vi "Teleop.vi"(10 "Match Info":T1={"Autonomous Elapsed Seconds"=0.0, "TeleOp Elapsed Seconds"=0.0, "Disabled Elapsed Seconds"=0.0, "Visited Autonomous"=FALSE, "Visited TeleOp"=FALSE, "Visited Disabled"=FALSE, "Autonomous Settings"={"Autonomous Style"=enum."Independent", "VI Refnum"=refnum}}, 11 "Call Context":T2) -> ()   [LabVIEW 2016]
doc: "This VI is called for each TeleOp packet received from the DS where the robot is not disabled. It is often used to read from the joysticks and update I/O or to update setpoints for timed control loops. It should complete and return within 20 milliseconds or it may miss DS packets."
uses:
  <vilib>/Rock Robotics/WPI/DriverStation/WPI_DriverStationDerivedRobotMode.ctl
  <vilib>/Rock Robotics/WPI/DriverStation/WPI_DriverStationMatch Info.ctl
  Refname/Controllers.ctl
  Refname/Motors.ctl
  Refname/Refname to String (Controllers).vi
  <vilib>/Rock Robotics/WPI/Utilities/WPI_GetSetVariantRefNum.vi
  Robot Global Data.vi
panel:
  out "Final Offsets":dbl[](array[numeric])
  out "error constant":errorcluster
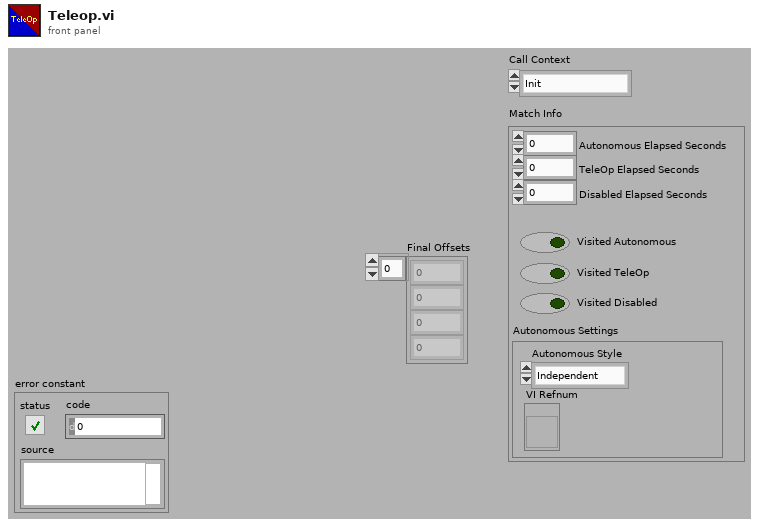
[diagram p1: front panel]
types:
  T1 = typedef "WPI_DriverStationMatch Info.ctl" = cluster{"Autonomous Elapsed Seconds":dbl, "TeleOp Elapsed Seconds":dbl, "Disabled Elapsed Seconds":dbl, "Visited Autonomous":bool, "Visited TeleOp":bool, "Visited Disabled":bool, "Autonomous Settings":cluster{"Autonomous Style":enum16{"Iterative", "Independent"}, "VI Refnum":refnum<vi>}}
  T2 = typedef "WPI_DriverStationDerivedRobotMode.ctl" = enum16{"Init", "Execute", "Stop"}
  T3 = cluster{"Joystick 1 X":dbl, "Joystick 1 Y":dbl, "Joystick 2 Z":dbl, "Joystick 2 Rotate":dbl}
  T4 = typedef "Controllers.ctl" = enum16{"Controller 0", "Controller 1"}
  T5 = typedef "Motors.ctl" = enum16{"Wheel 1", "Swerve 1", "Wheel 2", "Swerve 2", "Wheel 3", "Swerve 3", "Wheel 4", "Swerve 4"}
  T6 = cluster{"Encoder Offset 1":i32, "Encoder Offset 2":i32, "Encoder Offset 3":i32, "Encoder Offset 4":i32}
  T7 = typedef "WPI_JoystickDevRef.ctl" = cluster{"Device":T8}
  T8 = typedef "WPI_JoystickDeviceEnum.ctl" = enum16{"USB 0", "USB 1", "USB 2", "USB 3", "USB 4", "USB 5"}
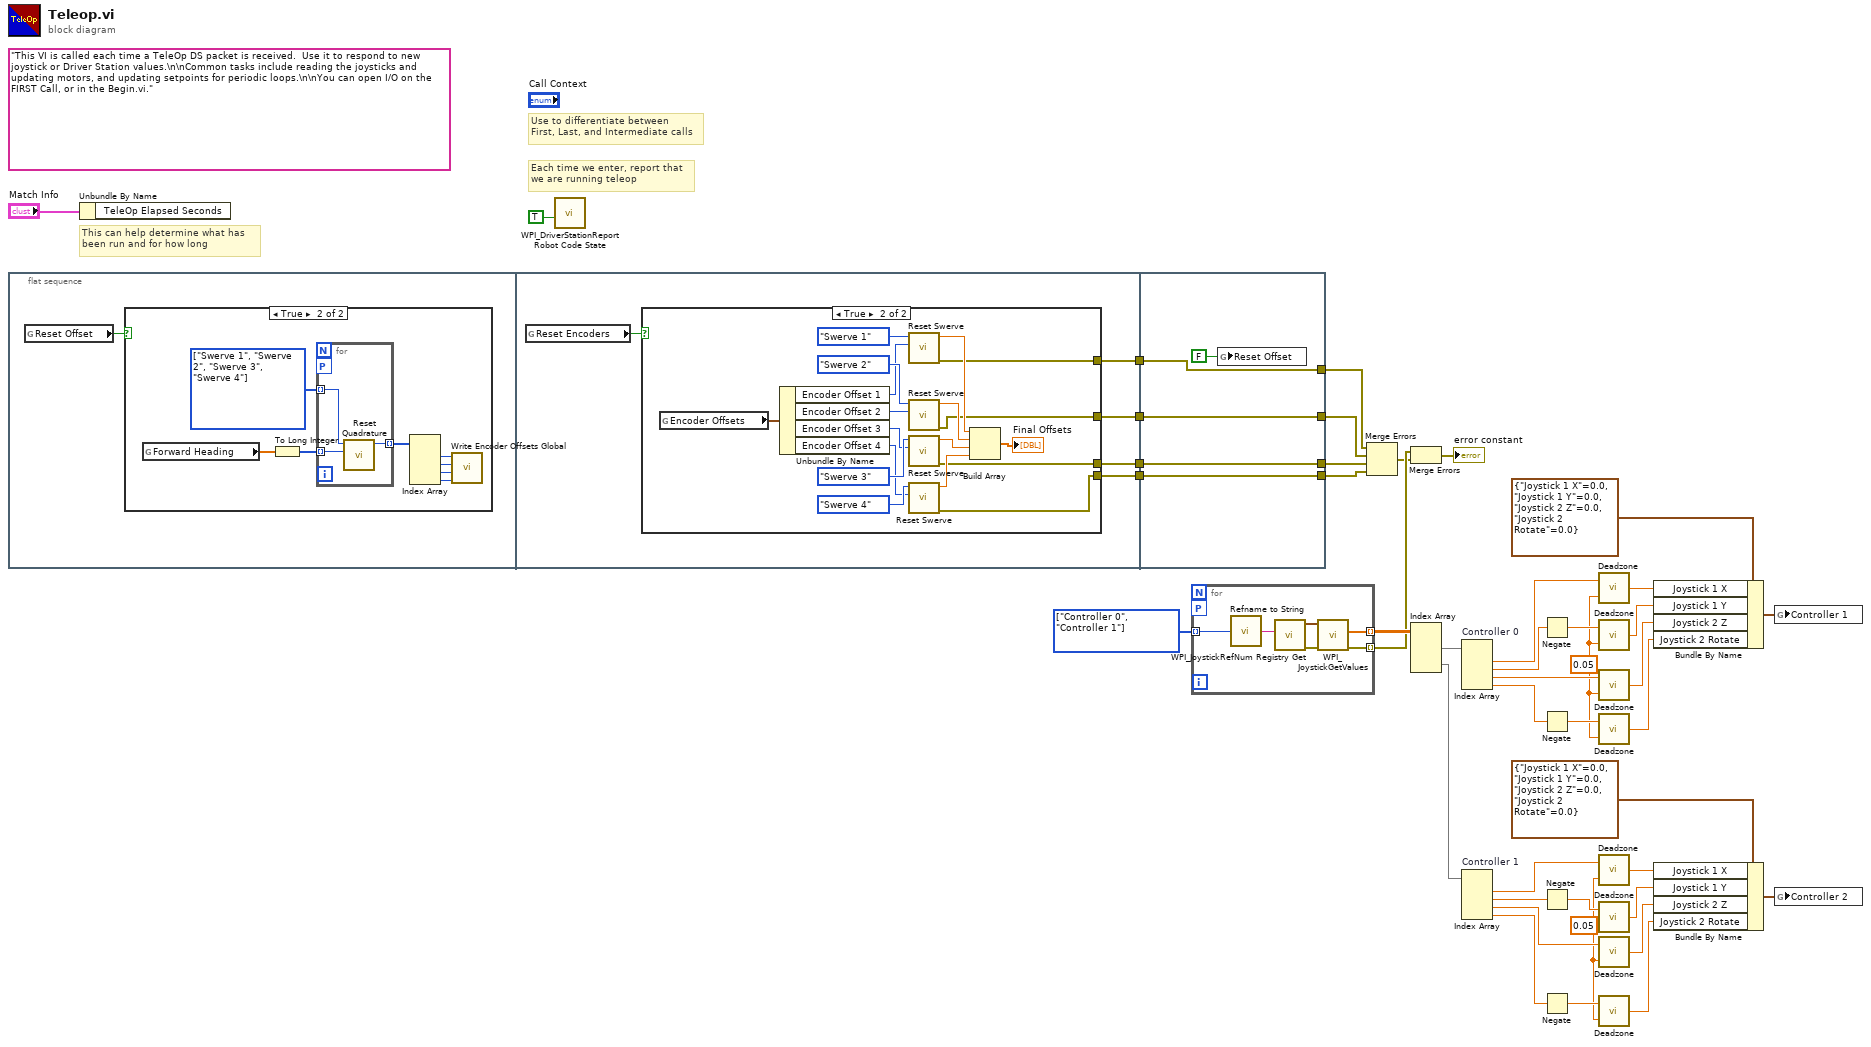
[diagram p0: block diagram]
diagram:
  w1 = 0.05
  w2 = 0.05
  w41 = T4[] [enum."Controller 0", enum."Controller 1"] items=["Controller 0", "Controller 1"]
  (unwired) "This VI is called each time a TeleOp DS packet is received.  Use it to respond to new joystick or Driver Station values.\n\nCommon tasks include reading the joysticks and updating motors, and updating setpoints for periodic loops.\n\nYou can open I/O on the FIRST Call, or in the Begin.vi."
  # "Each time we enter, report that\nwe are running teleop"
  # "Use to differentiate between\nFirst, Last, and Intermediate calls"
  # "This can help determine what has\nbeen run and for how long"
  n1 = flat-sequence {
    tunnel: [w59] -> w22
    tunnel: [w58] -> w21
    tunnel: [w57] -> w20
    tunnel: [w56] -> w19
    tunnel: [w80] -> w34
    tunnel: [w81] -> w35
    tunnel: [w82] -> w36
    tunnel: [w83] -> w37
    tunnel: w22 -> [w83]
    tunnel: w21 -> [w82]
    tunnel: w20 -> [w81]
    tunnel: w19 -> [w80]
    frame #0 {
      n2 = global read "Robot Global Data.vi" "Reset Offset"() -> (w44:bool)
      n3 = case shown="True" w44 {
        frame False {
        }
        frame True {
          w51 = T5[] [enum."Swerve 1", enum."Swerve 2", enum."Swerve 3", enum."Swerve 4"] items=["Wheel 1", "Swerve 1", "Wheel 2", "Swerve 2", "Wheel 3", "Swerve 3", "Wheel 4", "Swerve 4"]
          n4 = global read "Robot Global Data.vi" "Forward Heading"() -> (w49:dbl[])
          n5 = To Long Integer(number=w49) -> (32bit integer=w52:i32[])
          n6 = for {
            tunnel: w52 -> [w55] mode=indexing
            tunnel: w51 -> [w54] mode=indexing
            workers-P: _ -> [_]
            tunnel: [w53] -> w50 mode=indexing
            n7 = call "Reset Quadrature.vi"("Forward Position"=w55, "Enum"=w54) -> ("Encoder Offset"=w53:i32)  [unwired: 8 in, 1 out]
          }
          n8 = Index Array(array=w50) -> (element #1=w47:i32, element #2=w48:i32, element #3=w46:i32, element #4=w45:i32)  [unwired: 4 in]
          n9 = call "Write Encoder Offsets Global.vi"("Swerve 4"=w45, "Swerve 3"=w46, "Swerve 2"=w48, "Swerve 1"=w47) -> ()
        }
      }
    }
    frame #1 {
      n10 = global read "Robot Global Data.vi" "Reset Encoders"() -> (w60:bool)
      n11 = case shown="True" w60 {
        tunnel: [_ w69] -> w59
        tunnel: [_ w68] -> w58
        tunnel: [_ w67] -> w57
        tunnel: [_ w66] -> w56
        frame False {
        }
        frame True {
          n12 = global read "Robot Global Data.vi" "Encoder Offsets"() -> (w65:T6)
          n13 = Unbundle By Name(w65) -> ("Encoder Offset 1"=w64:i32, "Encoder Offset 2"=w63:i32, "Encoder Offset 3"=w62:i32, "Encoder Offset 4"=w61:i32)
          n14 = call "Reset Swerve.vi"("Encoder Offset"=w64, "Enum"=Motors."Swerve 1") -> ("error out"=w69:errorcluster, "Final Offset"=w74:dbl)  [unwired: 8 in]
          n15 = call "Reset Swerve.vi"("Encoder Offset"=w63, "Enum"=Motors."Swerve 2") -> ("error out"=w68:errorcluster, "Final Offset"=w73:dbl)  [unwired: 8 in]
          n16 = call "Reset Swerve.vi"("Encoder Offset"=w62, "Enum"=Motors."Swerve 3") -> ("error out"=w67:errorcluster, "Final Offset"=w72:dbl)  [unwired: 8 in]
          n17 = call "Reset Swerve.vi"("Encoder Offset"=w61, "Enum"=Motors."Swerve 4") -> ("error out"=w66:errorcluster, "Final Offset"=w71:dbl)  [unwired: 8 in]
          n18 = Build Array(w74, w73, w72, w71) -> (→"Final Offsets":dbl[])
        }
      }
    }
    frame #2 {
      n19 = global write "Robot Global Data.vi" "Reset Offset"(FALSE) -> ()
    }
  }
  n20 = Unbundle By Name("Match Info") -> ()  [unwired: 1 out]
  n21 = call <vilib>:"WPI_DriverStationReport Robot Code State.vi"("TeleOp"=TRUE ("Autonomous")) -> ()  [unwired: 10 in, 1 out]
  n22 = for {
    tunnel: w41 -> [w89] mode=indexing
    workers-P: _ -> [_]
    tunnel: [w86] -> w40 mode=indexing
    tunnel: [w85] -> w24 mode=indexing
    n23 = call-poly "Refname to String.vi"("Enum"=w89) -> ("string"=w88:string)
    n24 = call <vilib>:"WPI_JoystickRefNum Registry Get.vi"("refnum name"=w88) -> ("error out"=w84:errorcluster, "JoystickDevRef"=w87:T7)  [unwired: 9 in]
    n25 = call <vilib>:"WPI_JoystickGetValues.vi"("error in (no error)"=w84, "JoystickDevRef"=w87) -> ("error out"=w85:errorcluster, "Axes"=w86:dbl[])  [unwired: 5 in, 3 out]
  }
  n26 = Merge Errors(w37, w36, w35, w34) -> (w23:errorcluster)
  n27 = Merge Errors(w24, w23) -> (→"error constant":errorcluster)
  n28 = Index Array(array=w40) -> (element #1=w39:dbl[], element #2=w38:dbl[])  [unwired: 4 in]
  n29 = Index Array "Controller 0"(array=w39) -> (element #1=w18:dbl, element #2=w33:dbl, element #3=w14:dbl, element #4=w30:dbl)  [unwired: 4 in]
  n30 = Index Array "Controller 1"(array=w38) -> (element #1=w10:dbl, element #2=w29:dbl, element #3=w6:dbl, element #4=w28:dbl)  [unwired: 4 in]
  n31 = Negate(x=w33) -> (-x=w15:dbl)
  n32 = Negate(x=w30) -> (-x=w12:dbl)
  n33 = Negate(x=w29) -> (-x=w8:dbl)
  n34 = Negate(x=w28) -> (-x=w4:dbl)
  n35 = call "Deadzone.vi"("Deadzone"=w2, "Value"=w18) -> ("Numeric"=w17:dbl)
  n36 = call "Deadzone.vi"("Deadzone"=w2, "Value"=w15) -> ("Numeric"=w16:dbl)
  n37 = call "Deadzone.vi"("Deadzone"=w2, "Value"=w14) -> ("Numeric"=w13:dbl)
  n38 = call "Deadzone.vi"("Deadzone"=w2, "Value"=w12) -> ("Numeric"=w11:dbl)
  n39 = call "Deadzone.vi"("Deadzone"=w1, "Value"=w10) -> ("Numeric"=w9:dbl)
  n40 = call "Deadzone.vi"("Deadzone"=w1, "Value"=w8) -> ("Numeric"=w7:dbl)
  n41 = call "Deadzone.vi"("Deadzone"=w1, "Value"=w6) -> ("Numeric"=w5:dbl)
  n42 = call "Deadzone.vi"("Deadzone"=w1, "Value"=w4) -> ("Numeric"=w3:dbl)
  n43 = Bundle By Name(cluster=T3 {"Joystick 1 X"=0.0, "Joystick 1 Y"=0.0, "Joystick 2 Z"=0.0, "Joystick 2 Rotate"=0.0} ("input cluster"), "Joystick 1 X"=w17, "Joystick 1 Y"=w16, "Joystick 2 Z"=w13, "Joystick 2 Rotate"=w11) -> (w31:T3)
  n44 = Bundle By Name(cluster=T3 {"Joystick 1 X"=0.0, "Joystick 1 Y"=0.0, "Joystick 2 Z"=0.0, "Joystick 2 Rotate"=0.0} ("input cluster"), "Joystick 1 X"=w9, "Joystick 1 Y"=w7, "Joystick 2 Z"=w5, "Joystick 2 Rotate"=w3) -> (w26:T3)
  n45 = global write "Robot Global Data.vi" "Controller 1"(w31) -> ()
  n46 = global write "Robot Global Data.vi" "Controller 2"(w26) -> ()
